vi "Check if user ID in list.vi"(9 "User ID":string, 11 "User array":T3 {"Expire sec" format="%.2f"}) -> (1 "User access cluster":T1 {"Expire sec" format="%.2f"}, 2 "index":i32, 3 "In list?":bool)   [LabVIEW 2013]
doc: "Searches the User array list for the input \"User ID\". Case insensitive. If found, output \"In list?\" =T and user access cluster is returned."
uses:
  User Access Type defs/User access cluster array.ctl
  User Access Type defs/User access cluster.ctl
  User Access Type defs/Security level U8.ctl
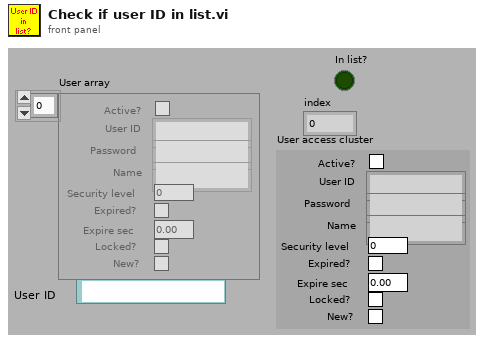
[diagram p1: front panel]
types:
  T1 = typedef "User access cluster.ctl" = cluster{"Active?":bool, "User ID":string, "Password":string, "Name":string, "Security level":T2, "Expired?":bool, "Expire sec":dbl, "Locked?":bool, "New?":bool}
  T2 = typedef "Security level U8.ctl" = u8
  T3 = typedef "User access cluster array.ctl" = T1[]
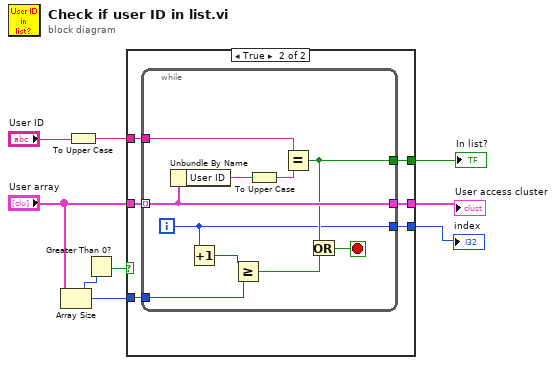
[diagram p0: block diagram]
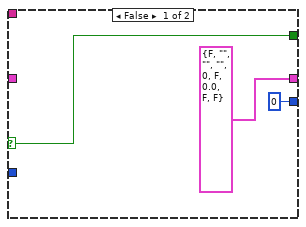
[diagram p2: hidden frame]
diagram:
  n1 = Array Size(array="User array") -> (size(s)=w3:i32)
  n2 = To Upper Case(1:"User ID") -> (0:w5:string)
  n3 = Greater Than 0?(x=w3) -> (x > 0?=w2:bool)
  n4 = case shown="True" w2 {
    selector: w2 -> [w11 _]
    tunnel: [T1 {"Active?"=FALSE, "User ID"="", "Password"="", "Name"="", "Security level"=0, "Expired?"=FALSE, "Expire sec"=0.0, "Locked?"=FALSE, "New?"=FALSE} ("User access cluster") w17] -> w8
    tunnel: "User array" -> [_ w16]
    tunnel: w5 -> [_ w15]
    tunnel: [w11 w14] -> w4
    tunnel: w3 -> [_ w13]
    tunnel: [0 w12] -> w1
    frame False {
    }
    frame True {
      n5 = while {
        tunnel: w16 -> [w27] mode=indexing
        tunnel: [w27] -> w17
        tunnel: w13 -> [w26]
        tunnel: w15 -> [w22]
        tunnel: [w19] -> w14
        tunnel: [w18] -> w12
        i -> [w18]
        stop <- w20 stop-if-true
        n6 = Unbundle By Name(w27) -> ("User ID"=w23:string)
        n7 = Increment(x=w18) -> (x+1=w25:i32)
        n8 = Greater Or Equal?(x=w25, y=w26) -> (x >= y?=w24:bool)
        n9 = To Upper Case(1:w23) -> (0:w21:string)
        n10 = Equal?(x=w22, y=w21) -> (x = y?=w19:bool)
        n11 = Or(x=w19, y=w24) -> (x .or. y?=w20:bool)
      }
    }
  }
  "In list?" <- w4
  "User access cluster" <- w8
  "index" <- w1
